vi "as UINT16.vi"(11 "bytes":u8[](array[numeric]) format="%b") -> (3 "UINT16":u16)   [LabVIEW 2020, in "MessagePack.lvlib" / "MessagePackNumeric.lvclass"]
uses:
  MessagePackNumeric.lvclass
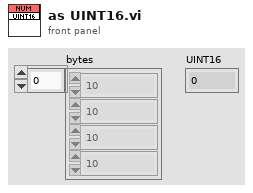
[diagram p1: front panel]
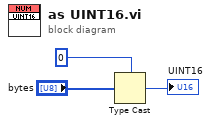
[diagram p0: block diagram]
diagram:
  n1 = Type Cast(type=u16 0 ("INT8"), x="bytes") -> (*(type *) &x=→"UINT16":u16)
